vi "Img_project_trapezoid.vi"(8 "error in (no error)":errorcluster, 11 "parameters":T1) -> (0 "error out":errorcluster, 3 "trapezoid_ROI":cluster{"X":dbl, "Y":dbl}[](array[cluster]))   [LabVIEW 2021, in "Framework_lib.lvlib"]
uses:
  QMH/Framework_lib.lvlib
panel:
  out "b":sgl
  out "m":sgl
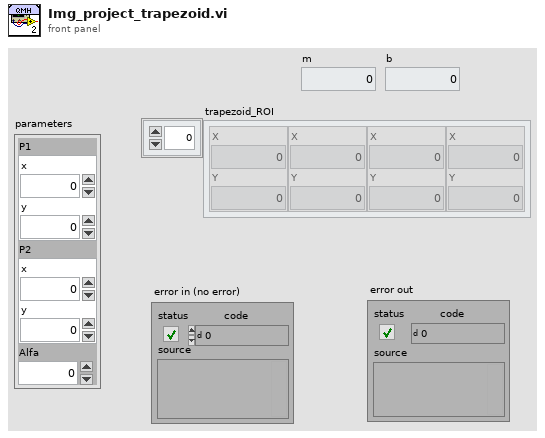
[diagram p1: front panel]
types:
  T1 = cluster{"P1":cluster{"x":i16, "y":i16}, "P2":cluster{"x":i16, "y":i16}, "Alfa":dbl}
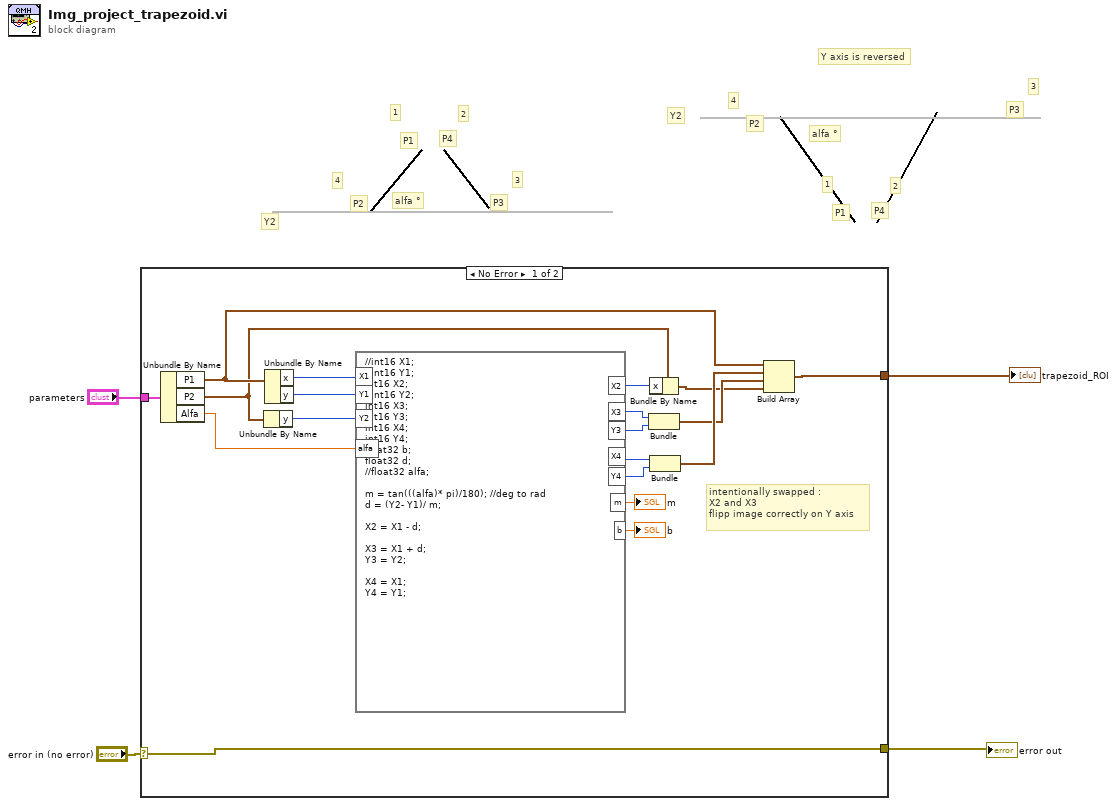
[diagram p0: block diagram]
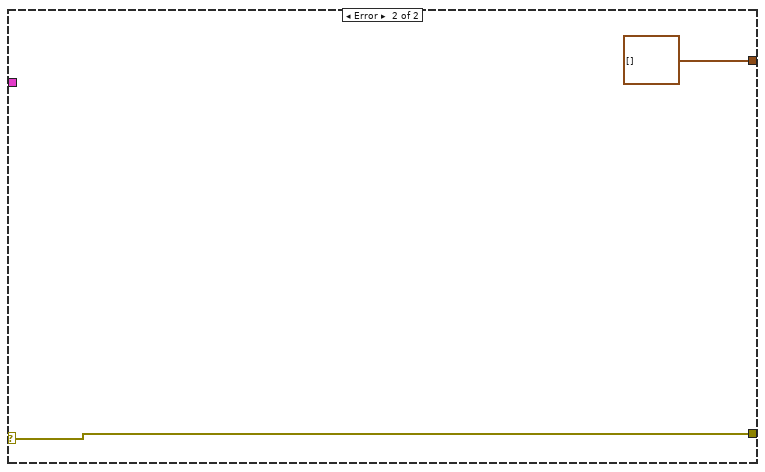
[diagram p2: hidden frame]
diagram:
  # "Y axis is reversed"
  # "alfa °"
  # "Y2"
  # "4"
  # "3"
  # "2"
  # "1"
  # "P4"
  # "P3"
  # "P2"
  # "P1"
  # "alfa °"
  # "Y2"
  # "4"
  # "3"
  # "2"
  # "1"
  # "P4"
  # "P3"
  # "P2"
  # "P1"
  n1 = case shown="No Error" "error in (no error)" {
    selector: "error in (no error)" -> [w11 w25]
    tunnel: [w12 cluster{"x":i16, "y":i16}[] []] -> w4
    tunnel: [w11 w25] -> w2
    tunnel: "parameters" -> [w10 _]
    frame No Error {
      # "intentionally swapped :\nX2 and X3\nflipp image correctly on Y axis"
      n2 = Unbundle By Name(w10) -> ("P1"=w9:cluster{"x":i16, "y":i16}, "P2"=w8:cluster{"x":i16, "y":i16}, "Alfa"=w7:dbl)
      n3 = Unbundle By Name(w8) -> ("y"=w21:i16)
      n4 = Unbundle By Name(w9) -> ("x"=w23:i16, "y"=w22:i16)
      n5 = formula code="//int16 X1;\n//int16 Y1;\nint16 X2;\n//int16 Y2;\nint16 X3;\nint16 Y3;\nint16 X4;\nint16 Y4;\nfloat32 b;\nfloat32 d;\n//float32 alfa;\n\nm = tan(((alfa)* pi)/180); //deg to rad\nd = (Y2- Y1)/ m;\n\nX2 = X1 - d;\n\nX3 = X1 + d;\nY3 = Y2;\n\nX4 = X1;\nY4 = Y1;"("X1"=w23, "Y1"=w22, "Y2"=w21, "alfa"=w7) -> ("X2"=w20:i16, "X3"=w19:i16, "Y3"=w18:i16, "X4"=w17:i16, "Y4"=w16:i16, "m"=→"m":dbl, "b"=→"b":sgl)
      n6 = Bundle(w19, w18) -> (w6:cluster{i16, i16})  [unwired: 1 in]
      n7 = Bundle By Name(cluster=w8, "x"=w20) -> (w5:cluster{"x":i16, "y":i16})
      n8 = Bundle(w17, w16) -> (w13:cluster{i16, i16})  [unwired: 1 in]
      n9 = Build Array(w9, w13, w6, w5) -> (w12:cluster{"x":i16, "y":i16}[])
    }
    frame Error {
    }
  }
  "error out" <- w2
  "trapezoid_ROI" <- w4
